vi "Least_squares.vi"() -> ()   [LabVIEW 2021]
uses:
  Globals/CH1.vi
  Globals/CH2.vi
  Globals/CH3.vi
  Globals/CH4.vi
  Globals/CH5.vi
  <vilib>/Analysis/NI_AALPro.lvlib
panel:
  in  "Y":enum16{"CH1", "CH2", "CH3", "CH4", "CH5"}(ring)=enum."CH2"
  in  "X":enum16{"CH1", "CH2", "CH3", "CH4", "CH5"}(ring)
  in  "WRITE":bool=TRUE
  out "d Ei [%]":dbl format="%#.2g"
  out "MAX (Y-(aX+b))":dbl format="%#.2g"
  out "MAX Y":dbl format="%#.2g"
  out "Y-(aX+b)":dbl[](array[numeric]) step=0.1 format="%#.3g"
  out "aX+b":dbl[](array[numeric]) step=0.1 format="%#.3g"
  out "SUM X":dbl format="%#.2g"
  out "SUM X*Y":dbl format="%#.2g"
  out "SUM Y":dbl format="%#.2g"
  out "SUM X":dbl format="%#.2g"
  out "X":dbl[](array[numeric]) step=0.1 format="%#.3g"
  out "X*Y":dbl[](array[numeric]) step=0.1 format="%#.3g"
  out "?":T1(graph)
  out "b":dbl format="%#_3g"
  out "a":dbl format="%#_3g"
  in  "Stop":bool
  in  "X                  Y":dbl[][](array[numeric]) step=0.1
  # "LEAST SQUARES METHOD"
  # "2"
  # "2"
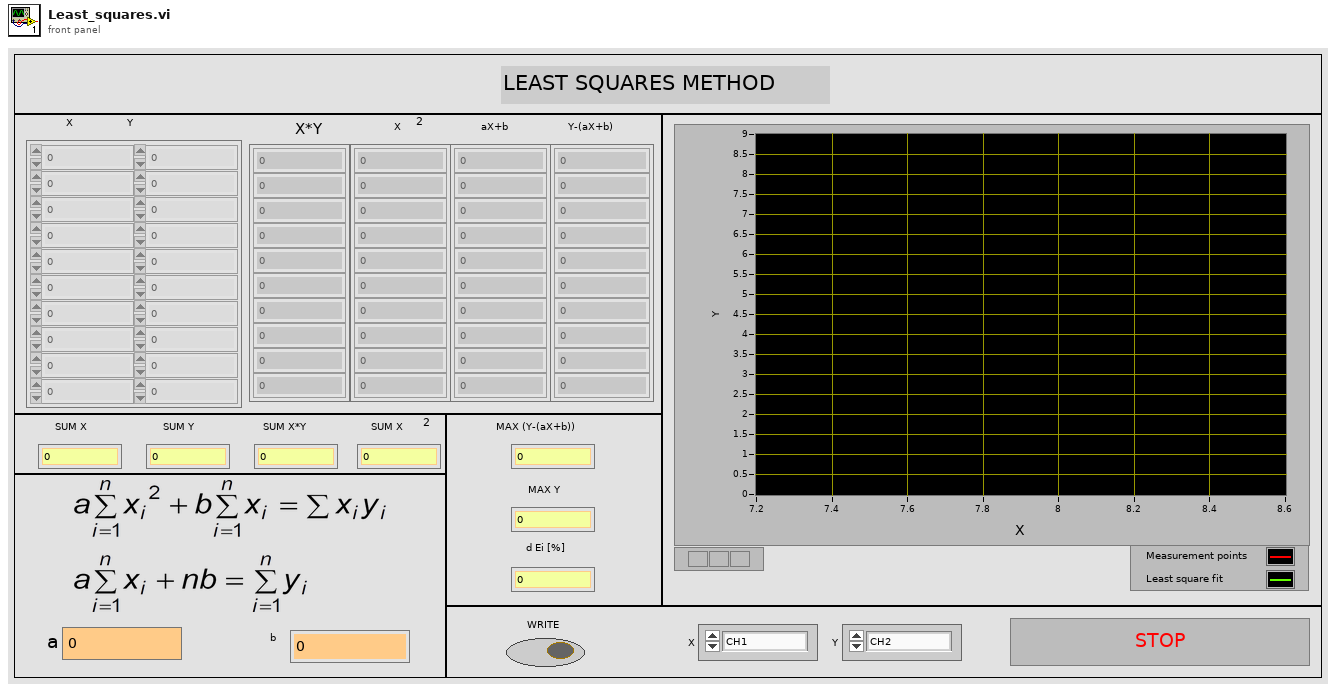
[diagram p1: front panel]
types:
  T1 = cluster{"Measured \nvalues":dbl[], "Measured \nvalues":dbl[]}[]
  T2 = cluster{"Measured \nvalues":dbl[], "Measured \nvalues":dbl[]}
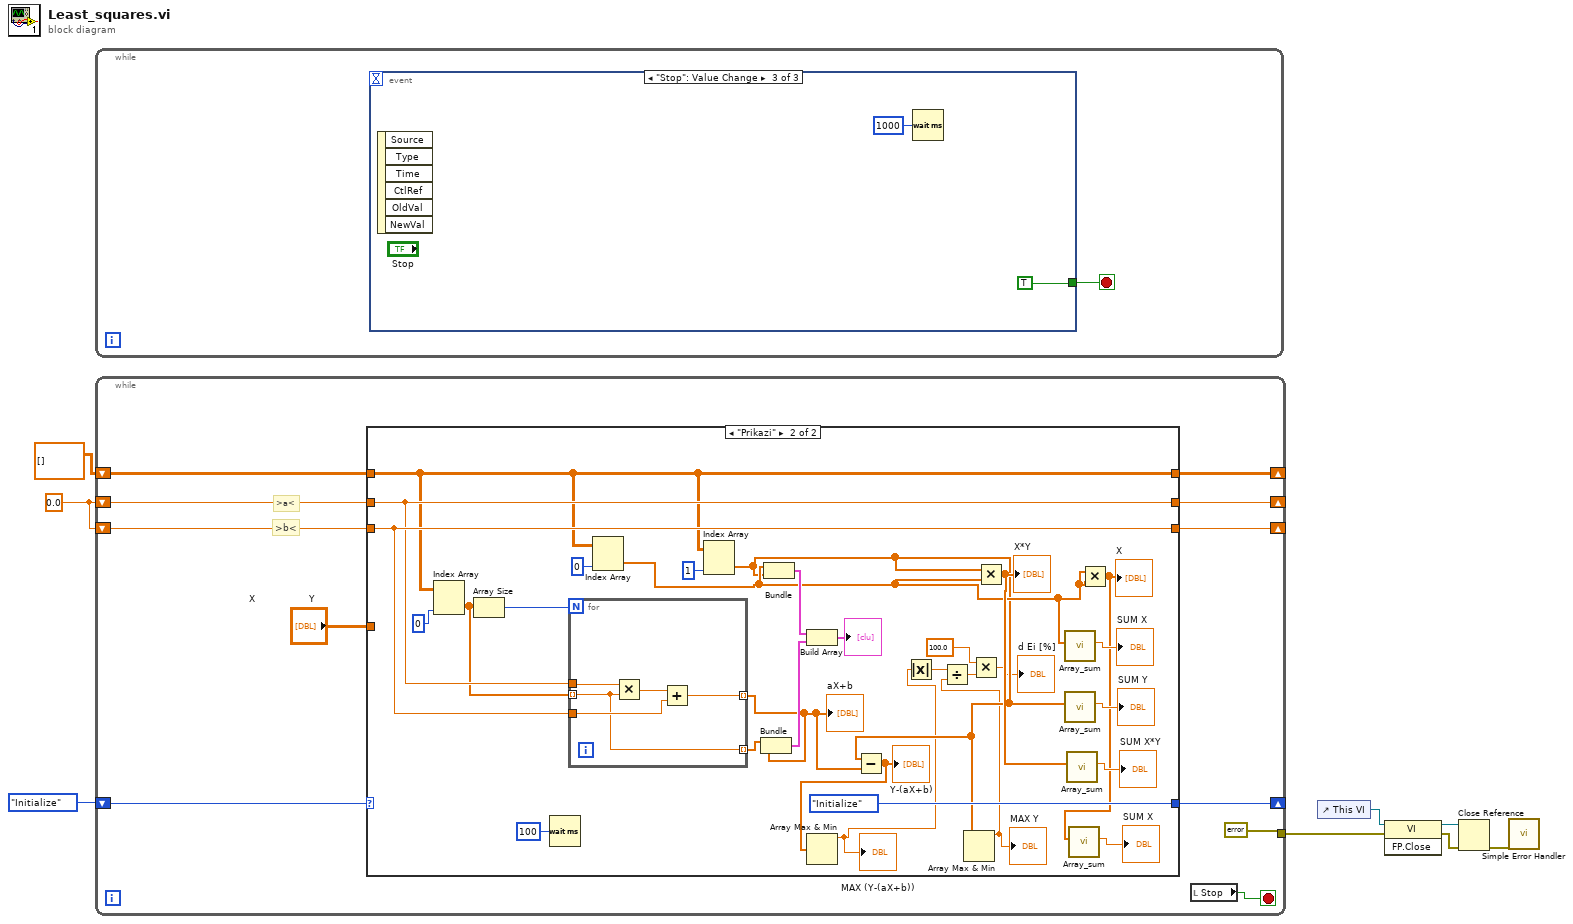
[diagram p0: block diagram]
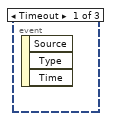
[diagram p2: hidden frame]
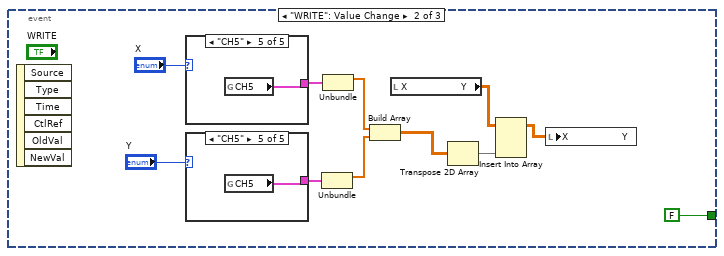
[diagram p3: hidden frame]
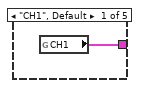
[diagram p4: hidden frame]
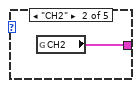
[diagram p5: hidden frame]
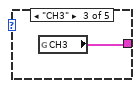
[diagram p6: hidden frame]
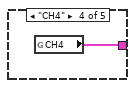
[diagram p7: hidden frame]
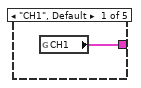
[diagram p8: hidden frame]
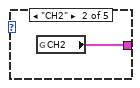
[diagram p9: hidden frame]
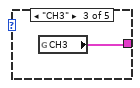
[diagram p10: hidden frame]
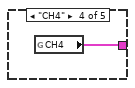
[diagram p11: hidden frame]
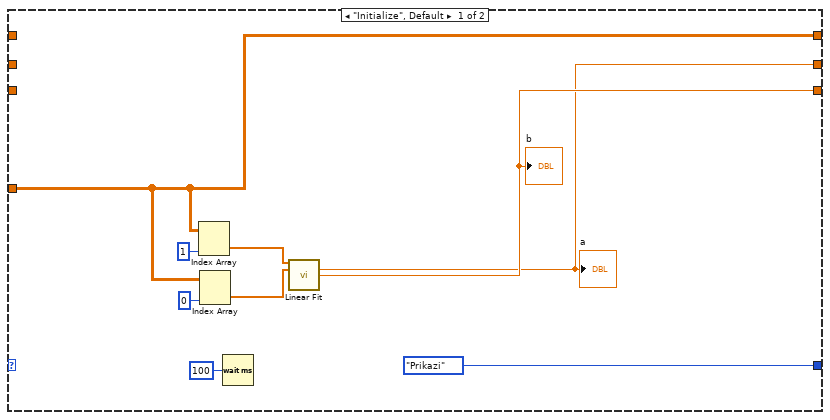
[diagram p12: hidden frame]
diagram:
  w7 = 0.0 ("Scalar")
  n1 = while {
    stop <- w9 stop-if-true
    n2 = event shown="[2] \"Stop\": Value Change" {
      selector: _ -> [_ _ _]
      dyn-events: _ -> [_ _ _]
      timeout: _ -> [_ _ _]
      tunnel: [_ FALSE TRUE] -> w9
      event Timeout {
        n3 = event-data() -> ()  [unwired: 1 in, 3 out]
      }
      event "WRITE": Value Change {
        n4 = event-data() -> ()  [unwired: 1 in, 6 out]
        n5 = case shown="\"CH5\"" "X" {
          tunnel: [w26 w27 w28 w29 w30] -> w18
          frame "CH1", Default {
            n6 = global read "CH1.vi" "CH1"() -> (w26:cluster{"CH1 Array":dbl[], "CH1 Message":string})
          }
          frame "CH2" {
            n7 = global read "CH2.vi" "CH2"() -> (w27:cluster{"CH2 Array":dbl[], "CH2 Message":string})
          }
          frame "CH3" {
            n8 = global read "CH3.vi" "CH3"() -> (w28:cluster{"CH3 Array":dbl[], "CH3 Message":string})
          }
          frame "CH4" {
            n9 = global read "CH4.vi" "CH4"() -> (w29:cluster{"CH4 Array":dbl[], "CH4 Message":string})
          }
          frame "CH5" {
            n10 = global read "CH5.vi" "CH5"() -> (w30:cluster{"CH5 Array":dbl[], "CH5 Message":string})
          }
        }
        n11 = case shown="\"CH5\"" "Y" {
          tunnel: [w21 w22 w23 w24 w25] -> w17
          frame "CH1", Default {
            n12 = global read "CH1.vi" "CH1"() -> (w21:cluster{"CH1 Array":dbl[], "CH1 Message":string})
          }
          frame "CH2" {
            n13 = global read "CH2.vi" "CH2"() -> (w22:cluster{"CH2 Array":dbl[], "CH2 Message":string})
          }
          frame "CH3" {
            n14 = global read "CH3.vi" "CH3"() -> (w23:cluster{"CH3 Array":dbl[], "CH3 Message":string})
          }
          frame "CH4" {
            n15 = global read "CH4.vi" "CH4"() -> (w24:cluster{"CH4 Array":dbl[], "CH4 Message":string})
          }
          frame "CH5" {
            n16 = global read "CH5.vi" "CH5"() -> (w25:cluster{"CH5 Array":dbl[], "CH5 Message":string})
          }
        }
        n17 = Unbundle(w17) -> ("CH5 Array"=w15:dbl[])  [unwired: 1 out]
        n18 = Unbundle(w18) -> ("CH5 Array"=w16:dbl[])  [unwired: 1 out]
        n19 = Build Array(w16, w15) -> (w12:dbl[][])
        n20 = local read "X                  Y"() -> (w14:dbl[][])
        n21 = Transpose 2D Array(2D array=w12) -> (transposed array=w11:dbl[][])
        n22 = Insert Into Array(array=w14, new element=w11) -> (w13:dbl[][])  [unwired: 2 in]
        n23 = local write "X                  Y"(w13) -> ()
      }
      event "Stop": Value Change {
        n24 = event-data() -> ()  [unwired: 1 in, 6 out]
        n25 = Wait (ms)(milliseconds to wait=u32 1000) -> ()  [unwired: 1 out]
      }
    }
  }
  n26 = while {
    shift-right: [w35] -> _
    shift-left: dbl[][] [] ("Measured \nvalues") -> [w42]
    shift-right: [w40] -> _
    shift-left: w7 -> [w37]
    shift-right: [w41] -> _
    shift-left: w7 -> [w36]
    shift-right: [w38] -> _
    shift-left: enum16{"Initialize", "Prikazi"}."Initialize" ("Enum") -> [w39]
    tunnel: [errorcluster {"status"=FALSE, "code"=0, "source"=""} ("error out")] -> w1
    stop <- w34 stop-if-true
    # ">b<"
    # ">a<"
    n27 = case shown="\"Prikazi\"" w39 {
      tunnel: "X                  Y" -> [w47 _]
      tunnel: [w47 w75] -> w35
      tunnel: w42 -> [_ w75]
      tunnel: [w45 w80] -> w41
      tunnel: [w44 w79] -> w40
      tunnel: [enum16{"Initialize", "Prikazi"}."Prikazi" ("Enum") enum16{"Initialize", "Prikazi"}."Initialize" ("Enum")] -> w38
      tunnel: w37 -> [_ w79]
      tunnel: w36 -> [_ w80]
      frame "Initialize", Default {
        n28 = Index Array(array=w47, index (col)=1 ("disabled index (col)")) -> (element=w48:dbl[])  [unwired: 1 in]
        n29 = Index Array(array=w47, index (col)=0 ("disabled index (col)")) -> (element=w46:dbl[])  [unwired: 1 in]
        n30 = Wait (ms)(milliseconds to wait=u32 100) -> ()  [unwired: 1 out]
        n31 = call <vilib>:"Linear Fit.vi"("Y"=w48, "X"=w46) -> ("slope"=w44:dbl, "intercept"=w45:dbl)  [unwired: 9 in, 3 out]
        "a" <- w44
        "b" <- w45
      }
      frame "Prikazi" {
        n32 = Index Array(array=w75, index (col)=0 ("disabled index (col)")) -> (element=w70:dbl[])  [unwired: 1 in]
        n33 = Array Size(array=w70) -> (size(s)=w71:i32)
        n34 = Wait (ms)(milliseconds to wait=u32 100) -> ()  [unwired: 1 out]
        n35 = for {
          N: w71 -> [_]
          tunnel: w80 -> [w85]
          tunnel: w79 -> [w87]
          tunnel: [w84] -> w60 mode=indexing
          tunnel: [w83] -> w63 mode=indexing
          tunnel: w70 -> [w83] mode=indexing
          n36 = Multiply(x=w87, y=w83) -> (x*y=w86:dbl)
          n37 = Add(x=w86, y=w85) -> (x+y=w84:dbl)
        }
        "aX+b" <- w60
        n38 = Index Array(array=w75, index (col)=0 ("disabled index (col)")) -> (element=w62:dbl[])  [unwired: 1 in]
        n39 = Index Array(array=w75, index (col)=1 ("disabled index (col)")) -> (element=w61:dbl[])  [unwired: 1 in]
        n40 = Bundle(w63, w60) -> (w73:cluster{dbl[], dbl[]})  [unwired: 1 in]
        n41 = Bundle("Measured \nvalues"=w62, "Measured \nvalues"=w61) -> (w74:T2)  [unwired: 1 in]
        n42 = Build Array(w74, w73) -> (→"?":T1)
        n43 = Subtract(x=w61, y=w60) -> (x-y=w59:dbl[])
        "Y-(aX+b)" <- w59
        n44 = Array Max & Min(array=w59) -> (max value=w57:dbl)  [unwired: 3 out]
        "MAX (Y-(aX+b))" <- w57
        n45 = Absolute Value(x=w57) -> (abs(x)=w58:dbl)
        n46 = Array Max & Min(array=w61) -> (max value=w56:dbl)  [unwired: 3 out]
        "MAX Y" <- w56
        n47 = Divide(x=w58, y=w56) -> (x/y=w55:dbl)
        n48 = Multiply(x=100.0, y=w55) -> (x*y=→"d Ei [%]":dbl)
        n49 = Multiply(x=w61, y=w62) -> (x*y=w66:dbl[])
        "X*Y" <- w66
        n50 = call "Array_sum.vi"("Array"=w62) -> ("Numeric"=→"SUM X":dbl)  [unwired: 10 in]
        n51 = call "Array_sum.vi"("Array"=w61) -> ("Numeric"=→"SUM Y":dbl)  [unwired: 10 in]
        n52 = call "Array_sum.vi"("Array"=w66) -> ("Numeric"=→"SUM X*Y":dbl)  [unwired: 10 in]
        n53 = Multiply(x=w62, y=w62) -> (x*y=w64:dbl[])
        "X" <- w64
        n54 = call "Array_sum.vi"("Array"=w64) -> ("Numeric"=→"SUM X":dbl)  [unwired: 10 in]
      }
    }
    n55 = local read "Stop"() -> (w34:bool)
  }
  n56 = control-ref of="This VI"() -> (w4:refnum<vi>)
  n57 = invoke class="VI" method="FP.Close"(reference=w4, error in=w1) -> (reference out=w2:refnum<vi>, error out=w3:errorcluster)  [unwired: 1 in, 1 out]
  n58 = Close Reference(reference=w2, error in (no error)=w3) -> (error out=w5:errorcluster)
  n59 = call <vilib>:"Simple Error Handler.vi"("error in (no error)"=w5) -> ()  [unwired: 4 in, 5 out]
